vi "AutoFeedForwardConversion.vi"(1 "Target Velocity (in/s)":dbl) -> (0 "Equivalent Joystick Command (ul)":dbl)   [LabVIEW 2020]
doc: "Converts the feed-forward path goal velocity from inches/sec to a unitless drive command. This VI is intended for use with the FRC 4265 Autonomous Path Planner and the pure-pursuit algorithm. The input is in inches per second and the output is a unitless equivalent joystick command."
uses:
  Globals/Calibration_And_Constant_Globals.vi
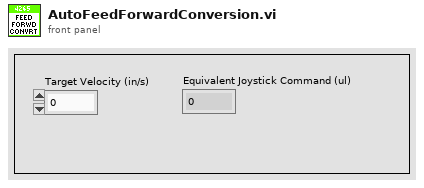
[diagram p1: front panel]
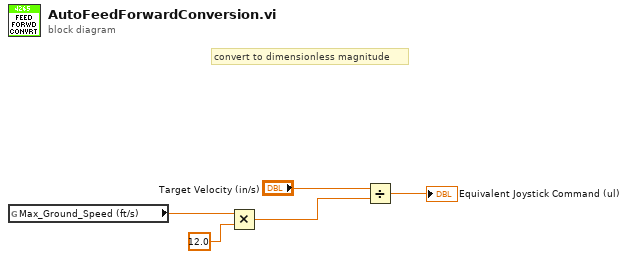
[diagram p0: block diagram]
diagram:
  # "convert to dimensionless magnitude"
  n1 = global read "Calibration_And_Constant_Globals.vi" "Max_Ground_Speed (ft/s)"() -> (w1:dbl)
  n2 = Multiply(x=w1, y=12.0) -> (x*y=w3:dbl)
  n3 = Divide(x="Target Velocity (in/s)", y=w3) -> (x/y=→"Equivalent Joystick Command (ul)":dbl)
